vi "Destroy.vi"(0 "reference":refnum<class "ArrowHead.lvclass">, 5 "error in (no error)":errorcluster) -> (19 "error out":errorcluster)   [LabVIEW 2016, in "ArrowHead.lvclass"]
doc: "Destroys an object created with a ArrowHead constructor VI or a subclass of the ArrowHead class. This VI must be reentrant.\n\n[GOOP 2.1]"
uses:
  <resource>/Framework/Providers/Open_GDS/UML/ArrowHead_class/ArrowHead.lvclass
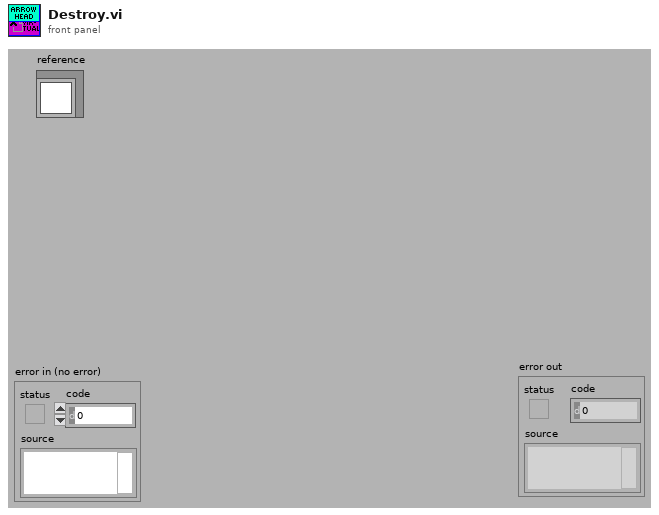
[diagram p1: front panel]
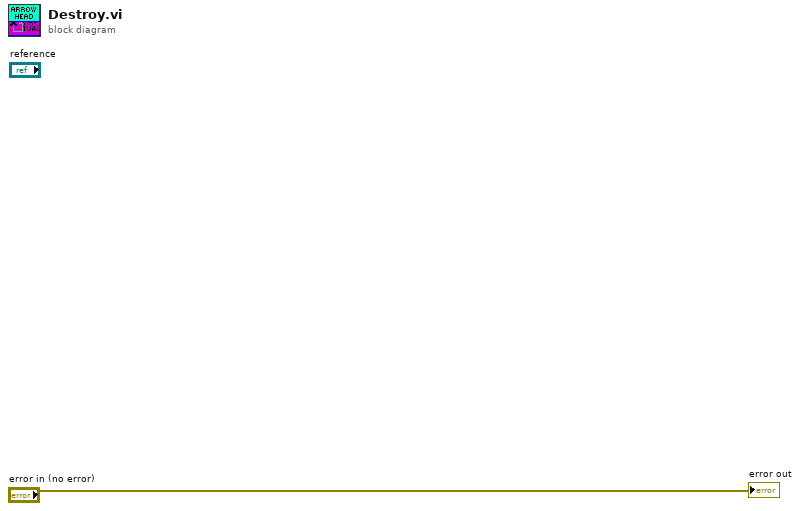
[diagram p0: block diagram]
diagram:
  "error out" <- "error in (no error)"
